vi "Sum 2D and Calc Centroid.vi"(11 "input array":i64[][](array[numeric])) -> (0 "Summed Array":i64[](array[numeric]), 1 "Index Array":i32[](array[numeric]), 3 "Centroid":dbl)   [LabVIEW 2013]
uses:
  <vilib>/Analysis/baseanly.llb/Real Dot Product.vi
  <vilib>/Analysis/NI_AALBase.lvlib
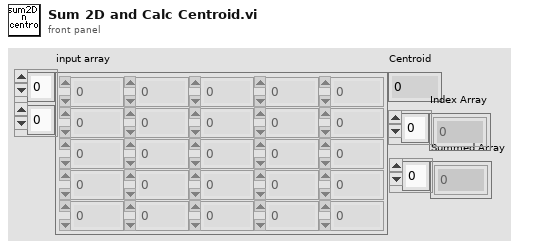
[diagram p1: front panel]
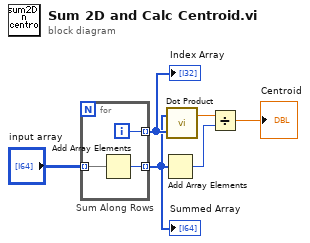
[diagram p0: block diagram]
diagram:
  n1 = for "Sum Along Rows" {
    tunnel: "input array" -> [w7] mode=indexing
    tunnel: [w9] -> w5 mode=indexing
    tunnel: [w8] -> w6 mode=indexing
    i -> [w8]
    n2 = Add Array Elements(numeric array=w7) -> (sum=w9:i64)
  }
  "Summed Array" <- w5
  "Index Array" <- w6
  n3 = Add Array Elements(numeric array=w5) -> (sum=w4:i64)
  n4 = call-poly <vilib>:"Dot Product.vi"("Y Vector"=w6, "X Vector"=w5) -> ("X * Y"=w3:dbl)  [unwired: 1 out]
  n5 = Divide(x=w3, y=w4) -> (x/y=→"Centroid":dbl)
